vi "GetSelectedTags.vi"(10 "Tree in":refnum<class "Tree.lvclass">) -> (0 "error out":errorcluster, 2 "Selected Tags":string[](array[string]), 3 "Tree out":refnum<class "Tree.lvclass">)   [LabVIEW 2021, in "Tree.lvlib" / "Tree.lvclass"]
uses:
  Tree.lvclass
  Tree.lvclass/Tree.ctl
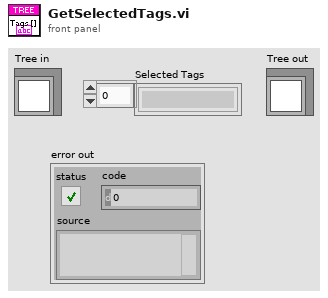
[diagram p1: front panel]
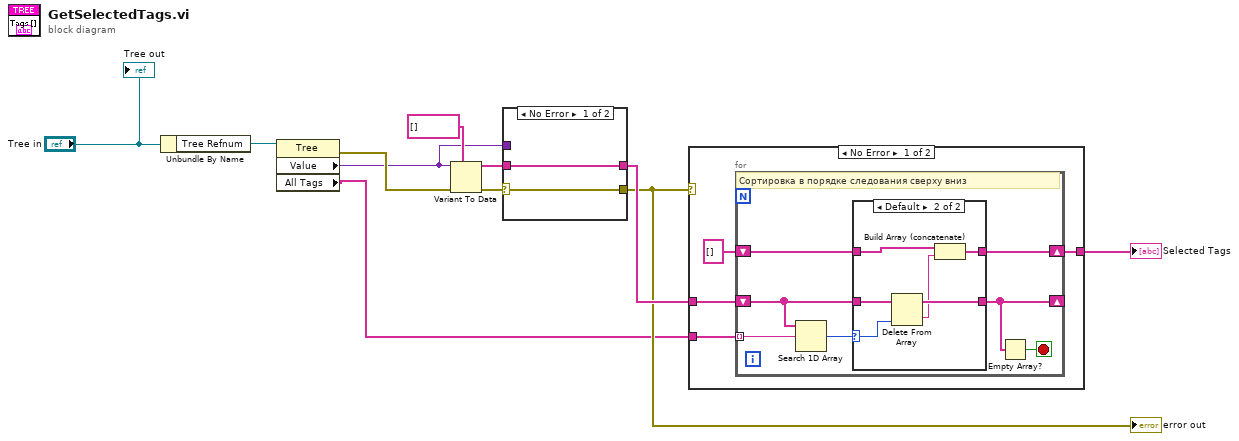
[diagram p0: block diagram]
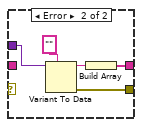
[diagram p4: hidden frame]
diagram:
  n1 = Unbundle By Name("Tree in") -> ("Tree Refnum"=w5:refnum<vi>)
  n2 = property class="Tree"(reference=w5) -> (error out=w7:errorcluster, "Value"=w6:variant, "All Tags"=w1:string[])  [unwired: 1 in, 1 out]
  n3 = Variant To Data(error in=w7, type=string[] [], Variant=w6) -> (data=w8:string[], error out=w9:errorcluster)
  n4 = case shown="No Error" w9 {
    selector: w9 -> [w13 _]
    tunnel: [w13 w17] -> w2
    tunnel: [w12 w15] -> w4
    tunnel: w8 -> [w12 _]
    tunnel: w6 -> [_ w14]
    frame No Error {
    }
    frame Error {
      n5 = Variant To Data(type="", Variant=w14) -> (data=w16:string, error out=w17:errorcluster)  [unwired: 1 in]
      n6 = Build Array(w16) -> (w15:string[])
    }
  }
  "error out" <- w2
  n7 = case shown="No Error" w2 {
    tunnel: w1 -> [w21 _]
    tunnel: w4 -> [w20 _]
    tunnel: [w19 _] -> w3
    frame No Error {
      n8 = for {
        tunnel: w21 -> [w29] mode=indexing
        shift-right: [w24] -> _
        shift-left: w20 -> [w28]
        shift-right: [w26] -> w19
        shift-left: string[] [] -> [w25]
        stop <- w23 stop-if-true
        # "Сортировка в порядке следования сверху вниз"
        n9 = Search 1D Array(1D array=w28, element=w29) -> (index of element=w27:i32)  [unwired: 1 in]
        n10 = case shown="Default" w27 {
          selector: w27 -> [_ w35]
          tunnel: w28 -> [w31 w37]
          tunnel: [w31 w36] -> w24
          tunnel: [w30 w33] -> w26
          tunnel: w25 -> [w30 w32]
          frame -1 {
          }
          frame Default {
            n11 = Delete From Array(array=w37, index=w35) -> (deleted portion=w34:string, array with subset deleted=w36:string[])  [unwired: 1 in]
            n12 = Build Array (concatenate)(w32, w34) -> (w33:string[])
          }
        }
        n13 = Empty Array?(array=w24) -> (empty?=w23:bool)
      }
    }
    frame Error {
    }
  }
  "Selected Tags" <- w3
  "Tree out" <- "Tree in"
